vi "init.vi"(8 "error in (no error)":errorcluster, 11 "controller in":refnum<class "controller.lvclass">) -> (0 "error out":errorcluster, 3 "controller out":refnum<class "controller.lvclass">)   [LabVIEW 2025, in "controller.lvclass"]
uses:
  controller.lvclass
  controller.lvclass/controller.ctl
  <vilib>/DAQmx/create/channels.llb/DAQmx Create Channel (AI-Temperature-Thermocouple).vi
  <vilib>/DAQmx/create/channels.llb/DAQmx Create Channel (DO-Digital Output).vi
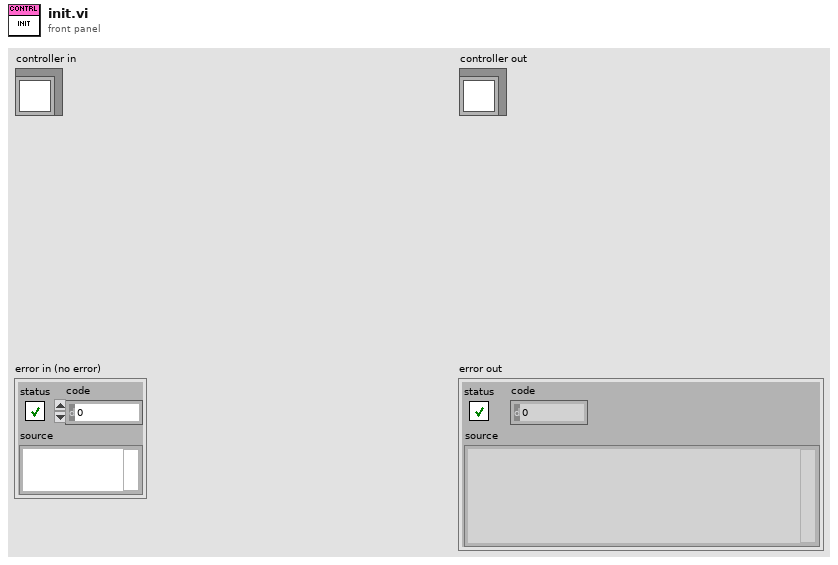
[diagram p1: front panel]
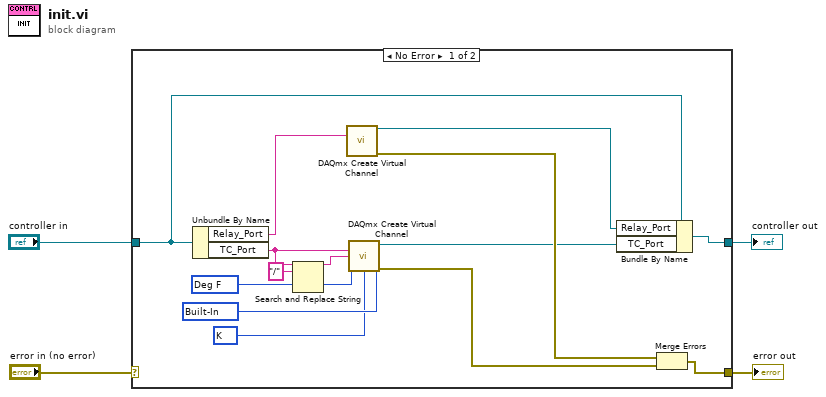
[diagram p0: block diagram]
diagram:
  n1 = case shown="No Error" "error in (no error)" {
    selector: "error in (no error)" -> [_ w20]
    tunnel: [w11 w20] -> w3
    tunnel: [w14 w19] -> w1
    tunnel: "controller in" -> [w13 w19]
    frame No Error {
      w15 = 10073 items=["J"=10072, "K"=10073, "N"=10077, "R"=10082, "S"=10085, "T"=10086, "B"=10047, "E"=10055] ("thermocouple type")
      w16 = 10200 items=["Built-In"=10200, "Constant Value"=10116, "Channel"=10113] ("cjc source")
      w17 = 10144 items=["Deg C"=10143, "Deg F"=10144, "Kelvins"=10325, "Deg R"=10145, "From Custom Scale"=10065] ("units")
      n2 = Unbundle By Name(w13) -> ("Relay_Port"=w18:string, "TC_Port"=w9:string)
      n3 = Search and Replace String(input string=w9, search string="/") -> (result string=w8:string)  [unwired: 6 in, 3 out]
      n4 = call-poly <vilib>:"DAQmx Create Virtual Channel.vi"("lines"=w18) -> ("task out"=w12:refnum<k21>, "error out"=w10:errorcluster)  [unwired: 13 in]
      n5 = call-poly <vilib>:"DAQmx Create Virtual Channel.vi"("physical channels"=w9, "cjc source"=w16, "name to assign"=w8, "units"=w17, "thermocouple type"=w15) -> ("task out"=w6:refnum<k21>, "error out"=w5:errorcluster)  [unwired: 9 in]
      n6 = Bundle By Name(cluster=w13, "Relay_Port"=w12, "TC_Port"=w6) -> (w14:refnum<class "controller.lvclass">)
      n7 = Merge Errors(w10, w5) -> (w11:errorcluster)
    }
    frame Error {
    }
  }
  "error out" <- w3
  "controller out" <- w1
